vi "Assert No Duplicate Named Private Data Elements.vi"(7 "class names":string[](array[string]), 8 "error in":errorcluster, 11 "private data clusters":variant[](array[variant])) -> (0 "error out":errorcluster)   [LabVIEW 2020, in "JKI JSON Object Serialization.lvlib" / "OOP_Utility.lvlib"]
uses:
  OOP_Utility.lvlib
  91249ab7-5ea3-4d6c-b8df-29db4c9f394f.vi
  f7c1a62c-1232-4a35-ba9e-0fa75d385864.vi
  91249ab7-5ea3-4d6c-b8df-29db4c9f394f.vi/73eff78f-802f-4e82-99e6-5ec6d44c8b1c.vi
  91249ab7-5ea3-4d6c-b8df-29db4c9f394f.vi/a79ef678-9021-4176-8e9d-ef71acec083e.vi
  91249ab7-5ea3-4d6c-b8df-29db4c9f394f.vi/6194b64b-8f19-4369-9ca4-18e99c56e175.vi
  91249ab7-5ea3-4d6c-b8df-29db4c9f394f.vi/4000f349-3ba7-45cd-93a4-b1a8967d5605.vi
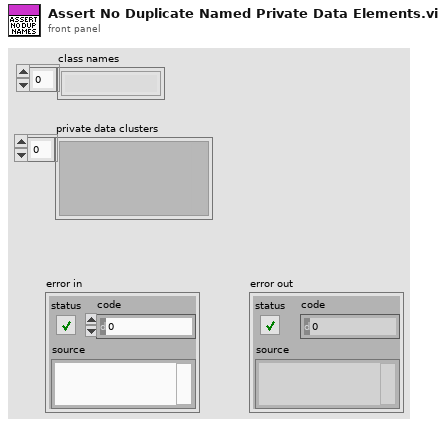
[diagram p1: front panel]
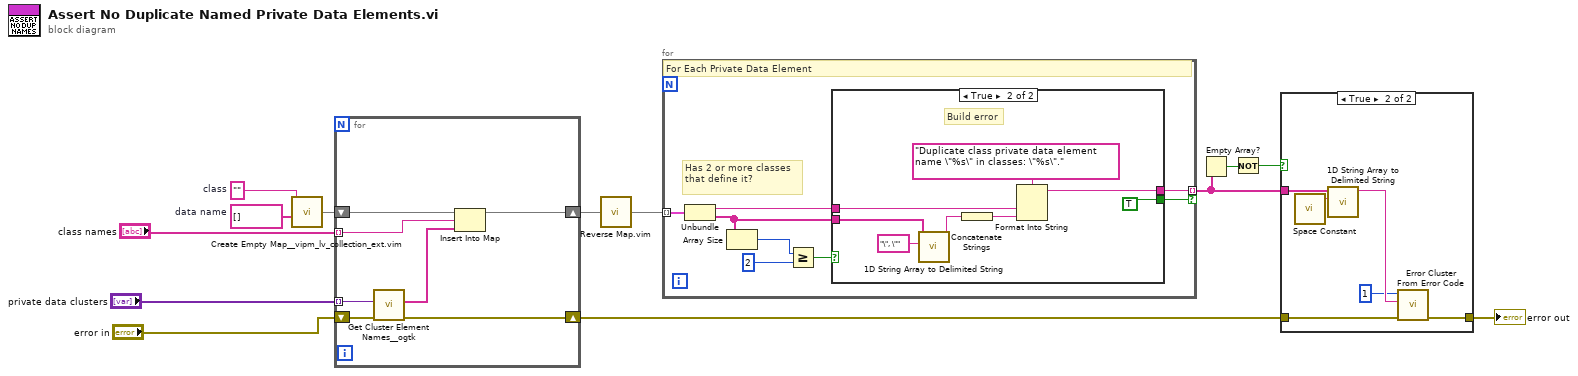
[diagram p0: block diagram]
diagram:
  w1 = string[] []  # data name
  w6 = ""  # class
  n1 = call "Create Empty Map__vipm_lv_collection_ext.vim"("value type"=w1, "key type"=w6) -> ("empty map"=w4:map{string, string[]})  [unwired: 8 in]
  n2 = for {
    tunnel: "private data clusters" -> [w14] mode=indexing
    shift-right: [w19] -> w12
    shift-left: "error in" -> [w20]
    tunnel: "class names" -> [w17] mode=indexing
    shift-right: [w16] -> w5
    shift-left: w4 -> [w18]
    n3 = call <userlib>:"Get Cluster Element Names__ogtk.vi"("error in (no error)"=w20, "Cluster"=w14) -> ("error out"=w19:errorcluster, "Element Names"=w15:string[])  [unwired: 8 in]
    n4 = Insert Into Map(map in=w18, key=w17, value=w15) -> (map out=w16:map{string, string[]})  [unwired: 2 out]
  }
  n5 = call "Reverse Map.vim"("map type (optional)"=w5) -> ("reversed map"=w8:map{string, string[]})  [unwired: 14 in]
  n6 = for {
    tunnel: w8 -> [w28] mode=indexing
    tunnel: [w22] -> w9 mode=indexing if=w21
    # "Has 2 or more classes that define it?"
    # "For Each Private Data Element"
    n7 = Unbundle(w28) -> ("key type"=w24:string, "value type"=w23:string[])
    n8 = Array Size(array=w23) -> (size(s)=w27:i32)
    n9 = Greater Or Equal?(x=w27, y=2) -> (x >= y?=w25:bool)
    n10 = case shown="True" w25 {
      tunnel: w24 -> [_ w36]
      tunnel: w23 -> [_ w30]
      tunnel: [_ w32] -> w22
      tunnel: [_ TRUE] -> w21
      frame False {
      }
      frame True {
        # "Build error"
        n11 = call <vilib>:"1D String Array to Delimited String.vi"("delimiter"="\", \"", "string array"=w30) -> ("delimited string"=w33:string)  [unwired: 9 in]
        n12 = Concatenate Strings(w33) -> (w29:string)
        n13 = Format Into String(format string="Duplicate class private data element name \"%s\" in classes: \"%s\".", w36, w29) -> (resulting string=w32:string)  [unwired: 2 in, 1 out]
      }
    }
  }
  n14 = Empty Array?(array=w9) -> (empty?=w10:bool)
  n15 = Not(x=w10) -> (.not. x?=w2:bool)
  n16 = case shown="True" w2 {
    tunnel: w9 -> [_ w42]
    tunnel: w12 -> [w37 w41]
    tunnel: [w37 w40] -> w13
    frame False {
    }
    frame True {
      n17 = call <vilib>:"Space Constant.vi"() -> ("String"=w43:string)
      n18 = call <vilib>:"1D String Array to Delimited String.vi"("delimiter"=w43, "string array"=w42) -> ("delimited string"=w39:string)  [unwired: 9 in]
      n19 = call <vilib>:"Error Cluster From Error Code.vi"("error in (no error)"=w41, "error message (\"\")"=w39, "error code (0)"=1) -> ("error out"=w40:errorcluster)  [unwired: 6 in]
    }
  }
  "error out" <- w13
